vi "Read SW version.vi"(6 "error in":errorcluster, 8 "MaxRead":i32, 9 "Channel in":u16) -> (0 "error out":errorcluster, 1 "SW Version":string, 2 "Pass":bool, 3 "Channel out":u16)   [LabVIEW 2023]
uses:
  143b1a18-0dc1-48a1-b4d9-00b0628c2b07.vi
  Communication/PCAN2023/PCAN API.lvlib
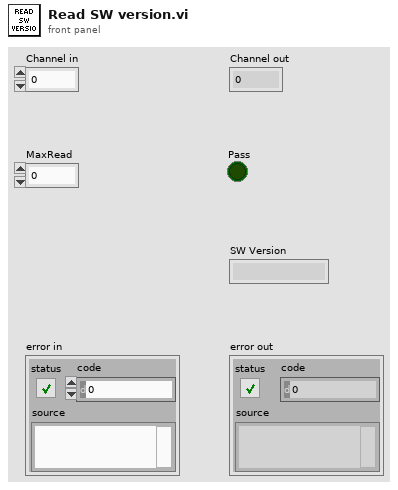
[diagram p1: front panel]
types:
  T1 = cluster{"ID":u32, "MSGTYPE":u8, "LEN":u8, "DATA[0]":u8, "DATA[1]":u8, "DATA[2]":u8, "DATA[3]":u8, "DATA[4]":u8, "DATA[5]":u8, "DATA[6]":u8, "DATA[7]":u8}
  T2 = cluster{"ID":u32, "MSGTYPE":u8, "LEN":u8, "DATA[0]":u8, "DATA[1]":u8, "DATA[2]":u8, "DATA[3]":u8, "DATA[4]":u8, "DATA[5]":u8, "DATA[6]":u8, "DATA[7]":u8}[]
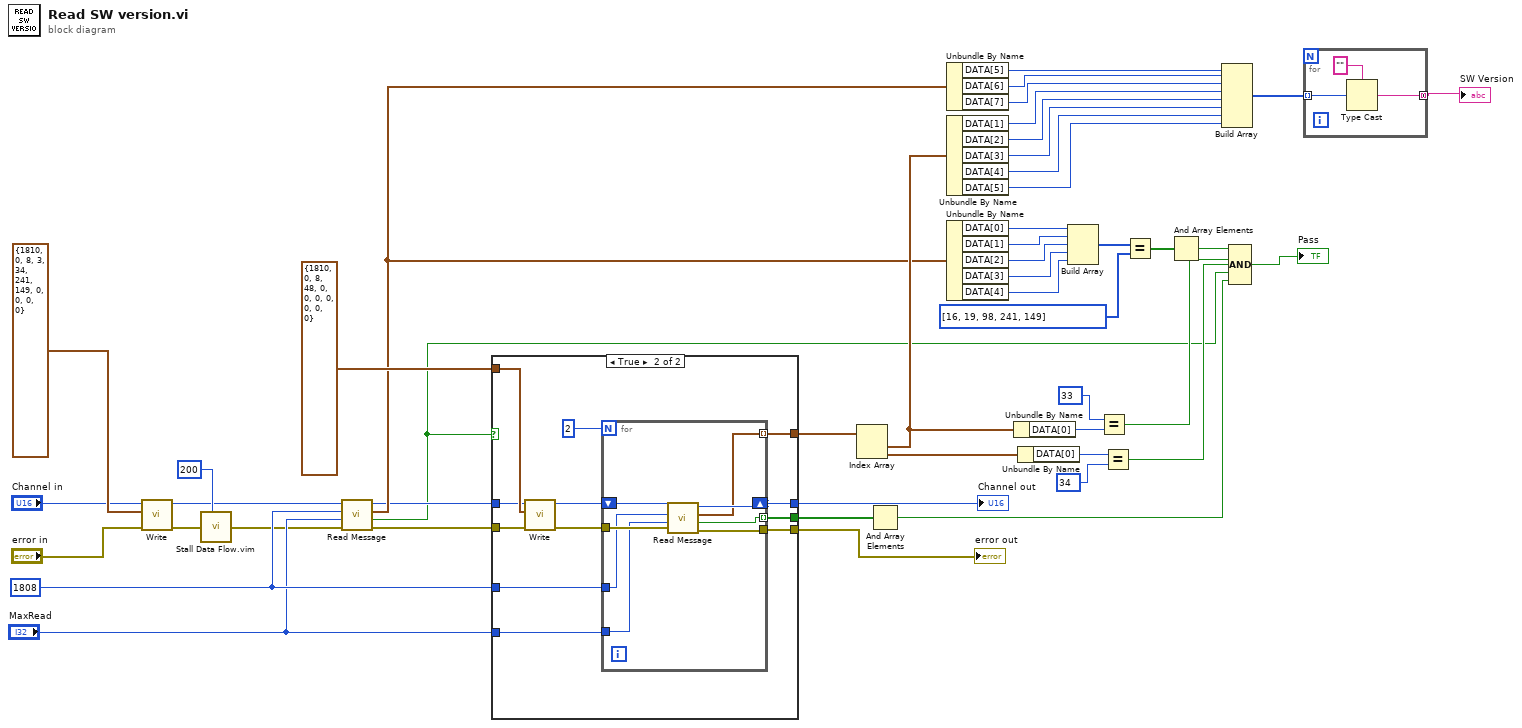
[diagram p0: block diagram]
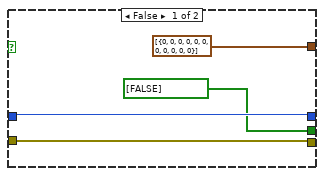
[diagram p2: hidden frame]
diagram:
  w7 = u32 1808 ("ID")
  n1 = call "Write.vi"("error in"="error in", "MessageBuffer"=T1 {"ID"=1810, "MSGTYPE"=0, "LEN"=8, "DATA[0]"=3, "DATA[1]"=34, "DATA[2]"=241, "DATA[3]"=149, "DATA[4]"=0, "DATA[5]"=0, "DATA[6]"=0, "DATA[7]"=0}, "Channel"="Channel in") -> ("error out"=w46:errorcluster, "Channel out"=w9:u16)  [unwired: 5 in, 2 out]
  n2 = call "Stall Data Flow.vim"("value in"=w46, "milliseconds to wait"=u32 200) -> ("value out"=w5:errorcluster)  [unwired: 1 out]
  n3 = call "Read Message.vi"("error in"=w5, "MaxRead"="MaxRead", "ID"=w7, "Channel in"=w9) -> ("error out"=w4:errorcluster, "Passed"=w1:bool, "Last Message"=w10:T1, "Channel out"=w8:u16)  [unwired: 3 in, 1 out]
  n4 = case shown="True" w1 {
    tunnel: T1 {"ID"=1810, "MSGTYPE"=0, "LEN"=8, "DATA[0]"=48, "DATA[1]"=0, "DATA[2]"=0, "DATA[3]"=0, "DATA[4]"=0, "DATA[5]"=0, "DATA[6]"=0, "DATA[7]"=0} ("MessageBuffer") -> [_ w63]
    tunnel: [T2 [{"ID"=0, "MSGTYPE"=0, "LEN"=0, "DATA[0]"=0, "DATA[1]"=0, "DATA[2]"=0, "DATA[3]"=0, "DATA[4]"=0, "DATA[5]"=0, "DATA[6]"=0, "DATA[7]"=0}] w59] -> w41
    tunnel: [w50 w58] -> w23
    tunnel: [w48 w57] -> w22
    tunnel: w8 -> [w50 w56]
    tunnel: w7 -> [_ w55]
    tunnel: "MaxRead" -> [_ w54]
    tunnel: w4 -> [w48 w53]
    tunnel: [bool[] [FALSE] w52] -> w3
    frame False {
    }
    frame True {
      n5 = call "Write.vi"("error in"=w53, "MessageBuffer"=w63, "Channel"=w56) -> ("error out"=w61:errorcluster, "Channel out"=w62:u16)  [unwired: 5 in, 2 out]
      n6 = for {
        N: 2 -> [_]
        tunnel: w61 -> [w69]
        tunnel: [w65] -> w59 mode=indexing
        shift-right: [w70] -> w58
        shift-left: w62 -> [w71]
        tunnel: [w68] -> w57
        tunnel: w55 -> [w67]
        tunnel: w54 -> [w66]
        tunnel: [w64] -> w52 mode=indexing
        n7 = call "Read Message.vi"("error in"=w69, "MaxRead"=w66, "ID"=w67, "Channel in"=w71) -> ("error out"=w68:errorcluster, "Passed"=w64:bool, "Last Message"=w65:T1, "Channel out"=w70:u16)  [unwired: 3 in, 1 out]
      }
    }
  }
  "error out" <- w22
  "Channel out" <- w23
  n8 = Index Array(array=w41) -> (element #1=w16:T1, element #2=w29:T1)  [unwired: 2 in]
  n9 = And Array Elements(Boolean array=w3) -> (logical AND=w2:bool)
  n10 = Unbundle By Name(w10) -> ("DATA[5]"=w21:u8, "DATA[6]"=w20:u8, "DATA[7]"=w19:u8)
  n11 = Unbundle By Name(w16) -> ("DATA[1]"=w15:u8, "DATA[2]"=w14:u8, "DATA[3]"=w13:u8, "DATA[4]"=w12:u8, "DATA[5]"=w11:u8)
  n12 = Unbundle By Name(w10) -> ("DATA[0]"=w40:u8, "DATA[1]"=w39:u8, "DATA[2]"=w38:u8, "DATA[3]"=w37:u8, "DATA[4]"=w36:u8)
  n13 = Unbundle By Name(w16) -> ("DATA[0]"=w33:u8)
  n14 = Unbundle By Name(w29) -> ("DATA[0]"=w30:u8)
  n15 = Build Array(w40, w39, w38, w37, w36) -> (w35:u8[])
  n16 = Equal?(x=u8 33, y=w33) -> (x = y?=w27:bool)
  n17 = Equal?(x=w30, y=u8 34 ("x")) -> (x = y?=w25:bool)
  n18 = Equal?(x=w35, y=u8[] [16, 19, 98, 241, 149]) -> (x = y?=w28:bool[])
  n19 = And Array Elements(Boolean array=w28) -> (logical AND=w26:bool)
  n20 = Build Array(w21, w20, w19, w15, w14, w13, w12, w11) -> (w18:u8[])
  n21 = Compound Arithmetic op=AND(w26, w27, w25, w1, w2) -> (→"Pass":bool)
  n22 = for {
    tunnel: w18 -> [w73] mode=indexing
    tunnel: [w72] -> w17 mode=concatenating
    n23 = Type Cast(type="", x=w73) -> (*(type *) &x=w72:string)
  }
  "SW Version" <- w17
